vi "PictureToImaq.vi"(8 "error in (no error)":errorcluster, 10 "Picture":picture, 11 "Image in":T1) -> (0 "error out":errorcluster, 3 "Image":T1)   [LabVIEW 2017]
uses:
  <vilib>/vision/Image Controls.llb/IMAQ Image.ctl
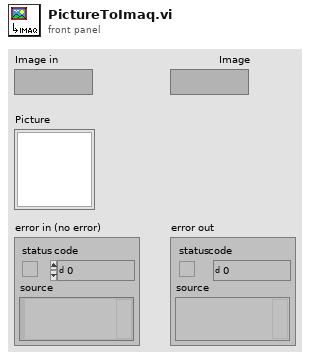
[diagram p1: front panel]
types:
  T1 = typedef "IMAQ Image.ctl" = refnum<image>
  T2 = typedef "imagedata.ctl" = cluster{"image type":i32, "image depth":i32, "image":u8[], "mask":u8[], "colors":u32[], "Rectangle":cluster{"left":i16, "top":i16, "right":i16, "bottom":i16}}
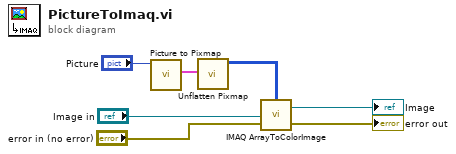
[diagram p0: block diagram]
diagram:
  n1 = call <vilib>:"Picture to Pixmap.vi"("picture"="Picture") -> ("image data"=w6:T2)  [unwired: 9 in, 1 out]
  n2 = call <vilib>:"Unflatten Pixmap.vi"("image data"=w6) -> ("24-bit pixmap"=w5:u32[][])  [unwired: 4 in, 6 out]
  n3 = call "IMAQ ArrayToColorImage"("Image Pixels (U32)"=w5, "Image"="Image in", "error in (no error)"="error in (no error)") -> ("Image Out"=→"Image":T1, "error out"=→"error out":errorcluster)  [unwired: 2 in]
